vi "LMS_FM_Demodulate_Example.vi"() -> ()   [LabVIEW 2013, in "LMS_LV_Drv.lvlib"]
uses:
  LMS_LV_Drv.lvlib
  Stream_ctl.ctl
  <vilib>/sound2/lvsound2.llb/Sampling Mode.ctl
  <vilib>/sound2/lvsound2.llb/Sound Data Format.ctl
  <vilib>/Analysis/3filter.llb/Filter Passband Type.ctl
  <vilib>/Analysis/1siggen.llb/Ramp Pattern by Samples.vi
  <vilib>/Analysis/2dsp.llb/Complex FFT.vi
  <vilib>/sound2/lvsound2.llb/Sound Output Write (DBL Single).vi
  <vilib>/Analysis/3filter.llb/Butterworth Filter (CDB).vi
  <vilib>/Analysis/2dsp.llb/Decimate (continuous, DBL).vi
  <vilib>/Analysis/NI_AALPro.lvlib
  <vilib>/Analysis/NI_AALBase.lvlib
panel:
  out "FM Spectrum":cluster{dbl[], dbl[]}[](graph)
  in  "Direction":u8(ring) items=["RX", "TX"]
  in  "Volume":dbl(knob)=0.8 min=0.0 max=2.0 step=0.1 scale=0.0..2.0
  in  "bandwidth":dbl=200000.0 format="%#_6p"
  out "EXIT":bool=TRUE
  in  "stop":bool
  in  "gain":u32=60
  in  "FM  Frequency":dbl(slide)=104300000.0 min=85000000.0 max=108000000.0 step=50000.0 scale=85000000.0..108000000.0 scale format="%#_6p"
  in  "chan":u64
  in  "stream":T1={"handle"=0, "isTx"=0, "channel"=0, "fifoSize"=100000, "throughputVsLatency"=1.0, "dataFmt"=0}
  out "LimeSDR_info":string="LimeSDR-USB, media=USB 3.0, module=FX3, serial=0009072C02891115, index=0"
  in  "Sample Rate":dbl=4000000.0 format="%#_6p"
  out "error out":errorcluster
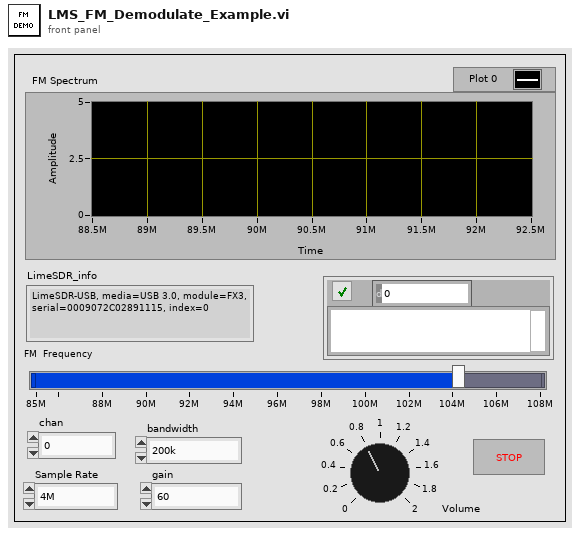
[diagram p1: front panel]
types:
  T1 = typedef "Stream_ctl.ctl" = cluster{"handle":u64, "isTx":u8, "channel":u32, "fifoSize":u32, "throughputVsLatency":dbl, "dataFmt":u32}
  T2 = typedef "Sound Data Format.ctl" = cluster{"sample rate (S/s)":dbl, "number of channels":i32, "bits per sample":i32}
  T3 = typedef "Sampling Mode.ctl" = i32
  T4 = typedef "Sound Output Task ID.ctl" = u32
  T5 = typedef "NI_AALBase.lvlib/Filter Passband Type.ctl" = enum32{"Lowpass", "Highpass", "Bandpass", "Bandstop"}
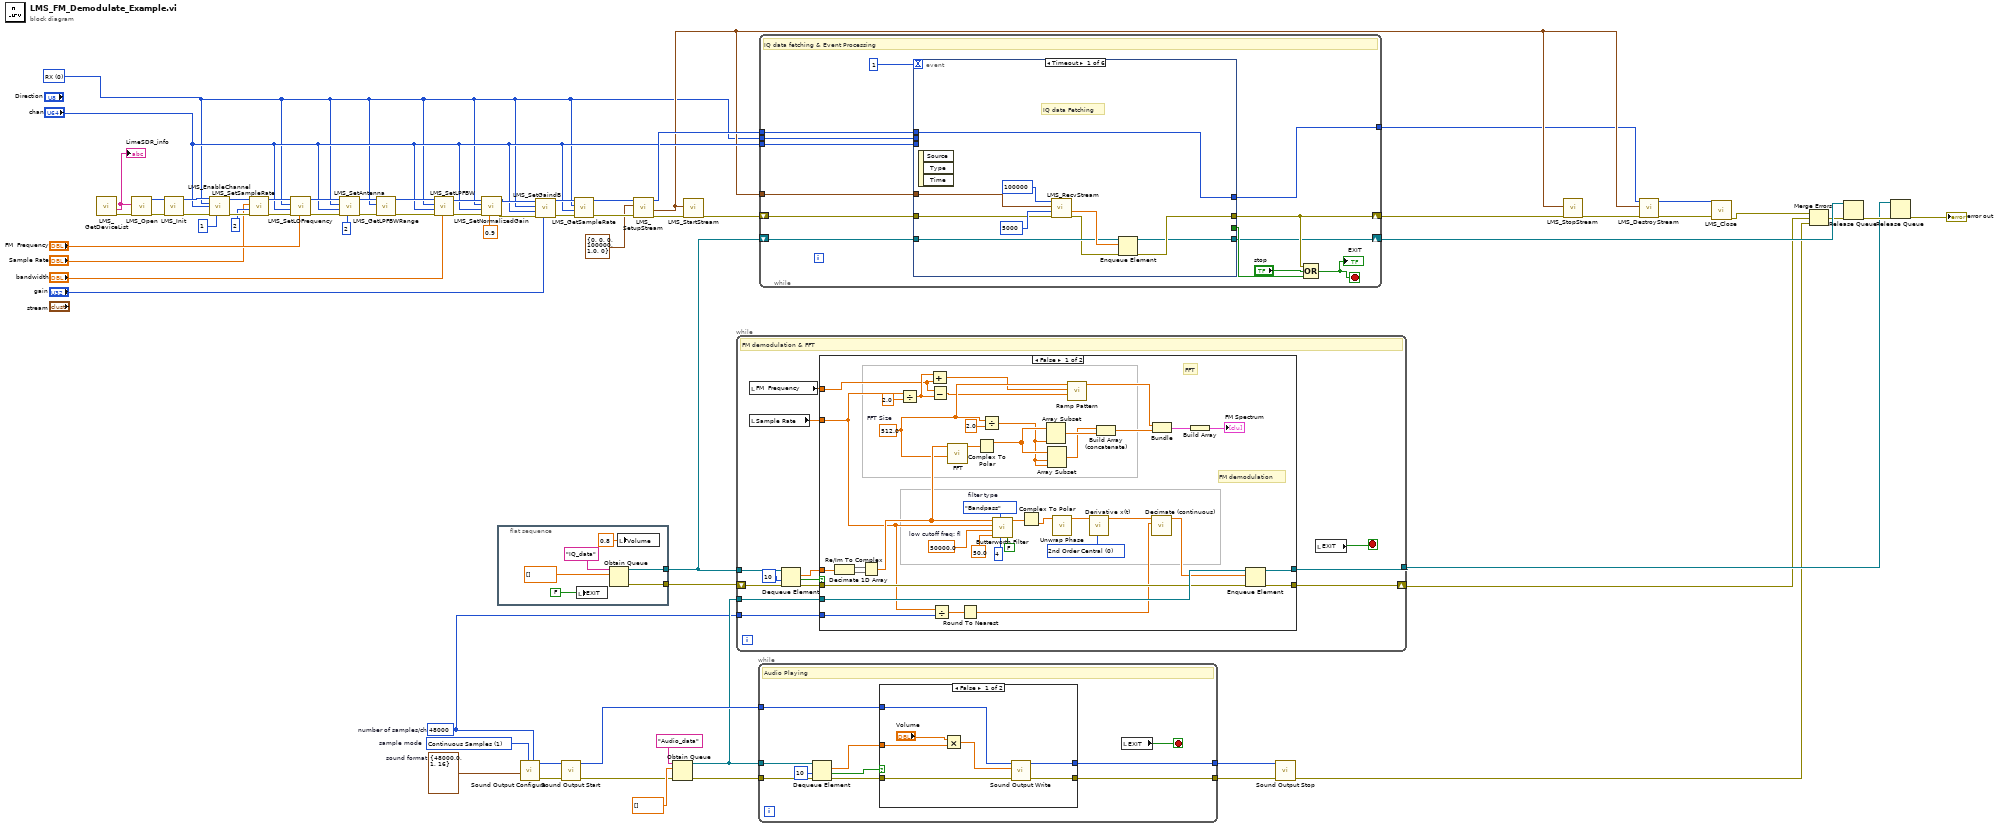
[diagram p0: block diagram]
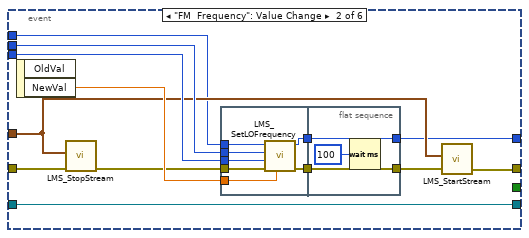
[diagram p4: hidden frame]
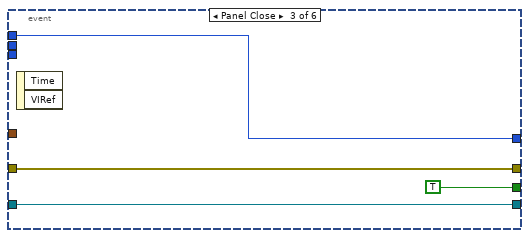
[diagram p5: hidden frame]
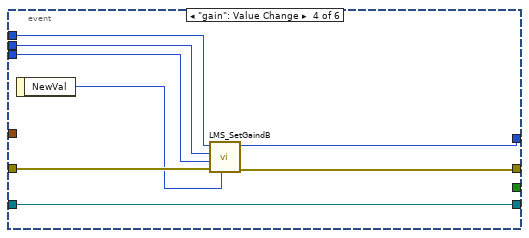
[diagram p6: hidden frame]
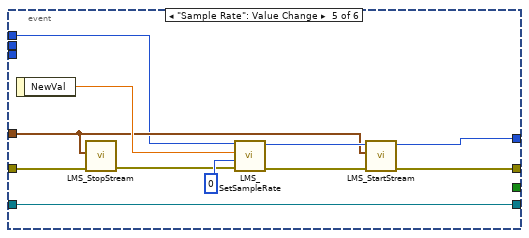
[diagram p7: hidden frame]
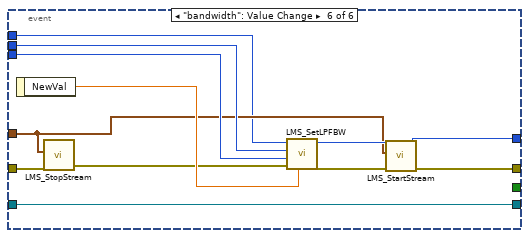
[diagram p8: hidden frame]
diagram:
  w6 = u8 0 items=["RX", "TX"] ("Direction")
  w4 = 48000  # number of samples/ch
  w30 = T2 {"sample rate (S/s)"=48000.0, "number of channels"=1, "bits per sample"=16}  # sound format
  w27 = T3 1 items=["Finite Samples", "Continuous Samples"]  # sample mode
  n1 = call "LMS_GetDeviceList.vi"() -> ("error out"=w67:errorcluster, "lms_info_str_t"=w66:string)  [unwired: 9 in, 1 out]
  "LimeSDR_info" <- w66
  n2 = call "LMS_Open.vi"("error in (no error)"=w67, "lms_info_str_t"=w66) -> ("error out"=w65:errorcluster, "device"=w64:i64)  [unwired: 8 in]
  n3 = call "LMS_Init.vi"("error in (no error)"=w65, "device_In"=w64) -> ("error out"=w54:errorcluster, "device_Out"=w55:i64)  [unwired: 8 in]
  n4 = call "LMS_EnableChannel.vi"("device_In"=w55, "dir_tx"=w6, "chan"="chan", "error in (no error)"=w54, "enabled"=i8 1) -> ("device_Out"=w51:i64, "error out"=w52:errorcluster)  [unwired: 9 in]
  n5 = call "LMS_SetSampleRate.vi"("error in (no error)"=w52, "oversample"=u64 2, "rate"="Sample Rate", "device_In"=w51) -> ("error out"=w50:errorcluster, "device_Out"=w49:i64)  [unwired: 6 in]
  n6 = call "LMS_SetLOFrequency.vi"("frequency"="FM  Frequency", "error in (no error)"=w50, "chan"="chan", "dir_tx"=w6, "device_In"=w49) -> ("error out"=w45:errorcluster, "device_Out"=w43:i64)  [unwired: 5 in]
  n7 = call "LMS_SetAntenna.vi"("index"=u64 2, "error in (no error)"=w45, "chan"="chan", "dir_tx"=w6, "device_In"=w43) -> ("error out"=w44:errorcluster, "device_Out"=w42:i64)  [unwired: 5 in]
  n8 = call "LMS_GetLPFBWRange.vi"("error in (no error)"=w44, "dir_tx"=w6, "device_In"=w42) -> ("error out"=w47:errorcluster, "device_Out"=w46:i64)  [unwired: 6 in, 1 out]
  n9 = call "LMS_SetLPFBW.vi"("bandwidth"="bandwidth", "error in (no error)"=w47, "chan"="chan", "dir_tx"=w6, "device_In"=w46) -> ("error out"=w40:errorcluster, "device_Out"=w57:i64)  [unwired: 5 in]
  n10 = call "LMS_SetNormalizedGain.vi"("gain"=0.9, "error in (no error)"=w40, "chan"="chan", "dir_tx"=w6, "device_In"=w57) -> ("error out"=w38:errorcluster, "device_Out"=w35:i64)  [unwired: 5 in]
  n11 = flat-sequence {
    tunnel: [w71] -> w36
    tunnel: [w68] -> w1
    frame #0 {
      n12 = local write "EXIT"(FALSE ("EXIT")) -> ()
      n13 = Obtain Queue(name (unnamed)="IQ_data", element data type=dbl[] [] ("samples")) -> (queue out=w71:refnum<queue>, error out=w68:errorcluster)  [unwired: 3 in, 1 out]
      n14 = local write "Volume"(0.8 ("Volume")) -> ()
    }
  }
  n15 = call <vilib>:"Sound Output Configure.vi"("number of samples/ch"=w4, "sample mode"=w27, "sound format"=w30) -> ("error out"=w28:errorcluster, "task ID"=w29:T4)  [unwired: 7 in]
  n16 = call "LMS_SetGaindB.vi"("gain"="gain", "error in (no error)"=w38, "chan"="chan", "dir_tx"=w6, "device_In"=w35) -> ("error out"=w18:errorcluster, "device_Out"=w17:i64)  [unwired: 5 in]
  n17 = call <vilib>:"Sound Output Start.vi"("error in (no error)"=w28, "task ID"=w29) -> ("error out"=w3:errorcluster, "task ID out"=w26:T4)  [unwired: 8 in]
  n18 = call "LMS_GetSampleRate.vi"("error in (no error)"=w18, "chan"="chan", "dir_tx"=w6, "device_In"=w17) -> ("error out"=w58:errorcluster, "device_Out"=w34:i64)  [unwired: 4 in, 2 out]
  n19 = call "LMS_SetupStream.vi"("error in (no error)"=w58, "stream_In"=T1 {"handle"=0, "isTx"=0, "channel"=0, "fifoSize"=100000, "throughputVsLatency"=1.0, "dataFmt"=0} ("stream"), "device_In"=w34) -> ("error out"=w63:errorcluster, "steam_Out"=w8:T1, "device_Out"=w10:i64)  [unwired: 6 in]
  n20 = Obtain Queue(name (unnamed)="Audio_data", element data type=dbl[] [] ("Decimated Array"), error in (no error)=w3) -> (queue out=w14:refnum<queue>, error out=w2:errorcluster)  [unwired: 2 in, 1 out]
  n21 = call "LMS_StartStream.vi"("error in (no error)"=w63, "stream 2"=w8) -> ("error out"=w11:errorcluster)  [unwired: 9 in]
  n22 = while {
    tunnel: w36 -> [w86]
    tunnel: w14 -> [w81]
    tunnel: [w80] -> w32
    shift-right: [w79] -> w22
    shift-left: w1 -> [w78]
    tunnel: w4 -> [w75]
    stop <- w83 stop-if-true
    # "FM demodulation & FFT"
    n23 = local read "FM  Frequency"() -> (w76:dbl)
    n24 = local read "Sample Rate"() -> (w74:dbl)
    n25 = Dequeue Element(queue=w86, timeout in ms (-1)=10, error in (no error)=w78) -> (element=w84:dbl[], timed out?=w85:bool, error out=w77:errorcluster)  [unwired: 1 out]
    n26 = case shown="False" w85 {
      tunnel: w84 -> [w124 _]
      tunnel: w74 -> [w87 _]
      tunnel: w81 -> [w118 w127]
      tunnel: [w117 w127] -> w80
      tunnel: [w116 w126] -> w79
      tunnel: w77 -> [w112 w126]
      tunnel: w76 -> [w93 _]
      tunnel: w75 -> [w89 _]
      frame False {
        w95 = 512.0  # FFT Size
        w119 = u16 0 items=["2nd Order Central", "4th Order Central", "Forward", "Backward"] ("method")
        w120 = Filter_Passband_Type."Bandpass"  # filter type
        w114 = 50000.0  # low cutoff freq: fl
        # "FFT"
        # "FM demodulation"
        n27 = Decimate 1D Array(w124) -> (w123:dbl[], w122:dbl[])
        n28 = Re/Im To Complex(1:w122, 2:w123) -> (0:w107:cdb[])
        n29 = Divide(x=w87, y=2.0) -> (x/y=w94:dbl)
        n30 = Add(x=w94, y=w93) -> (x+y=w91:dbl)
        n31 = Subtract(x=w93, y=w94) -> (x-y=w92:dbl)
        n32 = Divide(x=w87, y=w89) -> (x/y=w90:dbl)
        n33 = call-poly <vilib>:"FFT.vi"("FFT size"=w95, "X"=w107) -> ("FFT {X}"=w125:cdb[])  [unwired: 8 in, 1 out]
        n34 = Round To Nearest(number=w90) -> (nearest integer value=w88:dbl)
        n35 = Complex To Polar(r * e^(i*theta)=w125) -> (r=w103:dbl[])  [unwired: 1 out]
        n36 = Divide(x=w95, y=2.0) -> (x/y=w101:dbl)
        n37 = call-poly <vilib>:"Butterworth Filter.vi"("init/cont (init:F)"=FALSE, "order"=4, "filter type"=w120, "low cutoff freq: fl"=50.0, "high cutoff freq: fh"=w114, "sampling freq: fs"=w87, "X"=w107) -> ("Filtered X"=w106:cdb[])  [unwired: 1 in, 1 out]
        n38 = Complex To Polar(r * e^(i*theta)=w106) -> (theta=w111:dbl[])  [unwired: 1 out]
        n39 = Array Subset(array=w103, length=w101) -> (w105:dbl[])  [unwired: 1 in]
        n40 = Array Subset(array=w103, index=w101, length=w101) -> (w104:dbl[])
        n41 = call <vilib>:"Unwrap Phase.vi"("Phase"=w111) -> ("Unwrapped Phase"=w115:dbl[])  [unwired: 9 in, 1 out]
        n42 = call-poly <vilib>:"Ramp Pattern.vi"("start"=w92, "end"=w91, "samples"=w95) -> ("Ramp Pattern"=w96:dbl[])  [unwired: 7 in, 1 out]
        n43 = call <vilib>:"Derivative x(t).vi"("method"=w119, "X"=w115) -> ("dX/dt"=w110:dbl[])  [unwired: 8 in, 1 out]
        n44 = Build Array (concatenate)(w104, w105) -> (w98:dbl[])
        n45 = call-poly <vilib>:"Decimate (continuous).vi"("decimating factor"=w88, "X"=w110) -> ("Decimated Array"=w108:dbl[])  [unwired: 8 in, 1 out]
        n46 = Bundle("Ramp Pattern"=w96, w98) -> (w100:cluster{"Ramp Pattern":dbl[], dbl[]})  [unwired: 1 in]
        n47 = Build Array(w100) -> (→"FM Spectrum":cluster{"Ramp Pattern":dbl[], dbl[]}[])
        n48 = Enqueue Element(queue=w118, element=w108, error in (no error)=w112) -> (queue out=w117:refnum<queue>, error out=w116:errorcluster)  [unwired: 1 in, 1 out]
      }
      frame True {
      }
    }
    n49 = local read "EXIT"() -> (w83:bool)
  }
  n50 = while {
    tunnel: w14 -> [w135]
    tunnel: w26 -> [w133]
    tunnel: w2 -> [w129]
    tunnel: [w131] -> w25
    tunnel: [w130] -> w24
    stop <- w137 stop-if-true
    # "Audio Playing"
    n51 = Dequeue Element(queue=w135, timeout in ms (-1)=10, error in (no error)=w129) -> (element=w132:dbl[], timed out?=w134:bool, error out=w128:errorcluster)  [unwired: 1 out]
    n52 = case shown="False" w134 {
      tunnel: w133 -> [w141 w146]
      tunnel: w132 -> [w139 _]
      tunnel: w128 -> [w144 w145]
      tunnel: [w143 w145] -> w131
      tunnel: [w142 w146] -> w130
      frame False {
        n53 = Multiply(x="Volume", y=w139) -> (x*y=w140:dbl[])
        n54 = call-poly <vilib>:"Sound Output Write.vi"("error in (no error)"=w144, "data"=w140, "task ID"=w141) -> ("error out"=w143:errorcluster, "task ID out"=w142:T4)  [unwired: 7 in]
      }
      frame True {
      }
    }
    n55 = local read "EXIT"() -> (w137:bool)
  }
  n56 = while {
    tunnel: w8 -> [w155]
    shift-right: [w153] -> w59
    shift-left: w11 -> [w150]
    shift-right: [w147] -> w56
    shift-left: w36 -> [w148]
    tunnel: w10 -> [w159]
    tunnel: w6 -> [w158]
    tunnel: "chan" -> [w157]
    tunnel: [w156] -> w7
    stop <- w154 stop-if-true
    # "IQ data fetching & Event Processing"
    n57 = event shown="[0] Timeout" {
      selector: _ -> [_ _ _ _ _ _]
      dyn-events: _ -> [_ _ _ _ _ _]
      timeout: u32 1 ("milliseconds to wait") -> [_ _ _ _ _ _]
      tunnel: w150 -> [w166 w179 w196 w204 w211 w220]
      tunnel: w159 -> [w164 w170 w195 w202 w208 w216]
      tunnel: [w164 w175 w195 w201 w213 w224] -> w156
      tunnel: [w161 w178 w196 w203 w209 w218] -> w153
      tunnel: w158 -> [_ w182 _ w200 _ w223]
      tunnel: w157 -> [_ w181 _ w199 _ w222]
      tunnel: [_ _ TRUE _ _ _] -> w151
      tunnel: w155 -> [w165 w176 _ _ w210 w217]
      tunnel: w148 -> [w163 w177 w193 w197 w212 w221]
      tunnel: [w160 w177 w193 w197 w212 w221] -> w147
      event Timeout {
        # "IQ data Fetching"
        n58 = event-data() -> ()  [unwired: 1 in, 3 out]
        n59 = call "LMS_RecvStream.vi"("error in (no error)"=w166, "timeout_ms"=u32 5000, "stream"=w165, "sample_count"=u64 100000) -> ("error out"=w162:errorcluster, "samples"=w169:dbl[])  [unwired: 6 in]
        n60 = Enqueue Element(queue=w163, element=w169, error in (no error)=w162) -> (queue out=w160:refnum<queue>, error out=w161:errorcluster)  [unwired: 1 in, 1 out]
      }
      event "FM  Frequency": Value Change {
        n61 = event-data() -> ("NewVal"=w180:dbl)  [unwired: 1 in, 1 out]
        n62 = call "LMS_StopStream.vi"("error in (no error)"=w179, "stream"=w176) -> ("error out"=w171:errorcluster)  [unwired: 9 in]
        n63 = flat-sequence {
          tunnel: w182 -> [w189]
          tunnel: w181 -> [w188]
          tunnel: w180 -> [w187]
          tunnel: w171 -> [w186]
          tunnel: w170 -> [w185]
          tunnel: [w184] -> w173
          tunnel: [w183] -> w172
          tunnel: [w191] -> w174
          tunnel: [w192] -> w175
          tunnel: w173 -> [w192]
          tunnel: w172 -> [w191]
          frame #0 {
            n64 = call "LMS_SetLOFrequency.vi"("frequency"=w187, "error in (no error)"=w186, "chan"=w188, "dir_tx"=w189, "device_In"=w185) -> ("error out"=w183:errorcluster, "device_Out"=w184:i64)  [unwired: 5 in]
          }
          frame #1 {
            n65 = Wait (ms)(milliseconds to wait=u32 100) -> ()  [unwired: 1 out]
          }
        }
        n66 = call "LMS_StartStream.vi"("error in (no error)"=w174, "stream 2"=w176) -> ("error out"=w178:errorcluster)  [unwired: 9 in]
      }
      event Panel Close {
        n67 = event-data() -> ()  [unwired: 1 in, 2 out]
      }
      event "gain": Value Change {
        n68 = event-data() -> ("NewVal"=w198:u32)  [unwired: 1 in]
        n69 = call "LMS_SetGaindB.vi"("gain"=w198, "error in (no error)"=w204, "chan"=w199, "dir_tx"=w200, "device_In"=w202) -> ("error out"=w203:errorcluster, "device_Out"=w201:i64)  [unwired: 5 in]
      }
      event "Sample Rate": Value Change {
        n70 = event-data() -> ("NewVal"=w214:dbl)  [unwired: 1 in]
        n71 = call "LMS_StopStream.vi"("error in (no error)"=w211, "stream"=w210) -> ("error out"=w205:errorcluster)  [unwired: 9 in]
        n72 = call "LMS_SetSampleRate.vi"("error in (no error)"=w205, "oversample"=u64 0, "rate"=w214, "device_In"=w208) -> ("error out"=w206:errorcluster, "device_Out"=w213:i64)  [unwired: 6 in]
        n73 = call "LMS_StartStream.vi"("error in (no error)"=w206, "stream 2"=w210) -> ("error out"=w209:errorcluster)  [unwired: 9 in]
      }
      event "bandwidth": Value Change {
        n74 = event-data() -> ("NewVal"=w225:dbl)  [unwired: 1 in]
        n75 = call "LMS_StopStream.vi"("error in (no error)"=w220, "stream"=w217) -> ("error out"=w215:errorcluster)  [unwired: 9 in]
        n76 = call "LMS_SetLPFBW.vi"("bandwidth"=w225, "error in (no error)"=w215, "chan"=w222, "dir_tx"=w223, "device_In"=w216) -> ("error out"=w219:errorcluster, "device_Out"=w224:i64)  [unwired: 5 in]
        n77 = call "LMS_StartStream.vi"("error in (no error)"=w219, "stream 2"=w217) -> ("error out"=w218:errorcluster)  [unwired: 9 in]
      }
    }
    n78 = Compound Arithmetic op=OR(w153, "stop", w151) -> (w154:bool)
    "EXIT" <- w154
  }
  n79 = call <vilib>:"Sound Output Stop.vi"("error in (no error)"=w25, "task ID"=w24) -> ("error out"=w21:errorcluster)  [unwired: 8 in, 1 out]
  n80 = call "LMS_StopStream.vi"("error in (no error)"=w59, "stream"=w8) -> ("error out"=w60:errorcluster)  [unwired: 9 in]
  n81 = call "LMS_DestroyStream.vi"("error in (no error)"=w60, "stream"=w8, "device_In"=w7) -> ("error out"=w62:errorcluster, "device_Out"=w61:i64)  [unwired: 7 in]
  n82 = call "LMS_Close.vi"("error in (no error)"=w62, "device_In"=w61) -> ("error out"=w23:errorcluster)  [unwired: 9 in]
  n83 = Merge Errors(w23, w22, w21) -> (w20:errorcluster)
  n84 = Release Queue(queue=w56, error in (no error)=w20) -> (error out=w33:errorcluster)  [unwired: 1 in, 2 out]
  n85 = Release Queue(queue=w32, error in (no error)=w33) -> (error out=→"error out":errorcluster)  [unwired: 1 in, 2 out]
